vi "CSM - Mark As Worker Module.vi"(9 "CSM Name":string) -> (2 "CSM Name (Marked As Worker)":string)   [LabVIEW 2017, in "Communicable State Machine.lvlib"]
doc: "Marks a module as a Worker Mode module by adding `#` after the CSM name.\n\n<b>Reference Example</b>: `4. Advance Examples\\1. Action Workers Example`.\n\n\n> [!NOTE] <b>Name Concatenation API</b>\n>\n> This VI only manipulates the module name string and has no actual functionality. Therefore, once you are familiar with the CSM rules, you can directly enter name string and rule symbols without calling this API.\n\n\n> [!NOTE] <b>CSM Worker Mode</b>\n>\n> A CSM module implements Worker Mode by instantiating multiple instances, appending `#` to the requested name, and sharing the same message queue.\n> - From an external call perspective, these instances collectively form a composite module named Worker Agent.\n> - Each instance is named a Worker.\n>\n> <b>Behavior</b>: External callers can consider the Worker Agent as a single CSM module capable of message communication, state registration, and so on. Internally, an idle Worker retrieves messages from the Worker Agent message queue and processes them. Therefore, Worker Mode enables concurrent message processing for a CSM module.\n>\n> <b>Example</b>:\n>\n> // Request module name as `module#`, where `module` is the Worker Agent name. Instantiate two instances. Their names might be:\n> // - `module#59703F3AD837`\n> // - `module#106A470BA5EC`\n> // You cannot communicate directly with a Worker. You must communicate with the Worker Agent. For example:\n> `csm message >> arguments -@ module` // Synchronous message. An idle Worker will process this message.\n> `csm message >> arguments -> module` // Asynchronous message. An idle Worker will process this message.\n>\n> <b>Application Scenarios</b>:\n> - Call center operator scenarios\n> - Concurrent downloader scenarios\n> - Concurrent compiler scenarios\n> - TCP Server handling multiple Client connections\n\n\n-- <b>Controls</b> --\n- <b>CSM Name</b>: CSM module name.\n\n-- <b>Indicators</b> --\n- <b>CSM Name (Marked As Worker)</b>: CSM module name marked with `#`."
uses:
  Communicable State Machine.lvlib
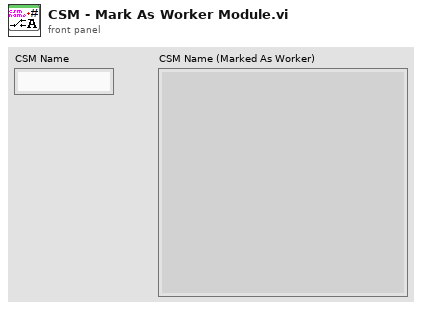
[diagram p1: front panel]
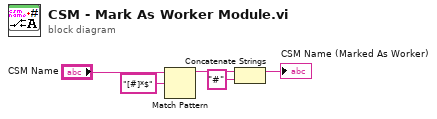
[diagram p0: block diagram]
diagram:
  n1 = Match Pattern(string="CSM Name", regular expression="[#]*$") -> (before substring=w3:string)  [unwired: 1 in, 3 out]
  n2 = Concatenate Strings(w3, "#" ("string")) -> (→"CSM Name (Marked As Worker)":string)
